vi "MRC Ds Comms Control Write Ansi.vi"(8 "error in (no error)":errorcluster, 11 "text":T1) -> (0 "error out":errorcluster)   [LabVIEW 2026, in "MrcLib.lvlib"]
doc: "MRC_Status MRC_CALLCONV MRC_DsCommsControl_WriteAnsi(const struct MRC_String* text);"
uses:
  MrcLib.lvlib
  MrcLib.dll
  Types/MRC String.ctl
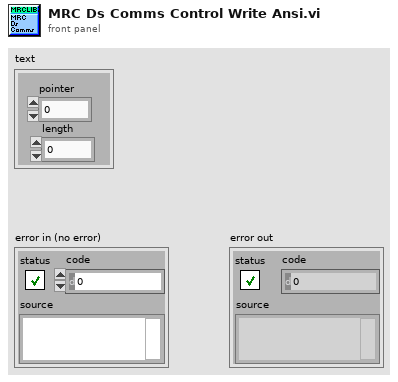
[diagram p1: front panel]
types:
  T1 = typedef "MRC String.ctl" = cluster{"pointer":u64, "length":u64}
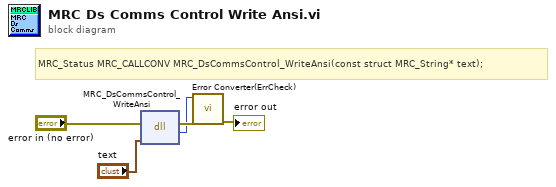
[diagram p0: block diagram]
diagram:
  # "MRC_Status MRC_CALLCONV MRC_DsCommsControl_WriteAnsi(const struct MRC_String* text);"
  n1 = dll-call lib="MrcLib.*" fn="MRC_DsCommsControl_WriteAnsi"(error in="error in (no error)", "text"="text") -> (error out=w3:errorcluster, "return type"=w1:i32)  [unwired: 3 in, 1 out]
  n2 = call "Error Converter(ErrCheck).vi"("error in (no error)"=w3, "status"=w1) -> ("error out"=→"error out":errorcluster)  [unwired: 9 in]
